vi "NavX.vi"(8 "error in":errorcluster) -> ()   [LabVIEW 2015]
uses:
  navx-mxp/labview/navX-MXP Library/COMMON/TypeDefs/Data TypeDefs/navX YPRH Data.ctl
  navx-mxp/labview/navX-MXP Library/COMMON/TypeDefs/Value TypeDefs/navX Interface Protocol.ctl
  <vilib>/Rock Robotics/SystemInterfaces/i2clib/i2c_bus.ctl
  LED Lights/LED Lights Global.vi
  <vilib>/Rock Robotics/Network Tables/NT Write Number.vi
  navx-mxp/labview/navX-MXP Library/navX-MXP IMU.lvlib
panel:
  out "Yaw":dbl
  out "YPRH":T1
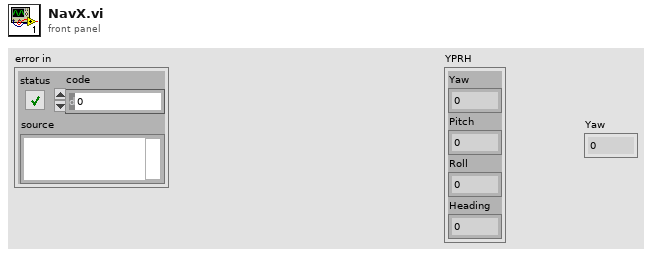
[diagram p1: front panel]
types:
  T1 = typedef "navX-MXP IMU.lvlib/navX YPRH Data.ctl" = cluster{"Yaw":dbl, "Pitch":dbl, "Roll":dbl, "Heading":dbl}
  T2 = typedef "i2c_bus.ctl" = enum16{"I2C On-Board", "I2C MXP", "Invalid"}
  T3 = typedef "navX-MXP IMU.lvlib/navX Interface Protocol.ctl" = enum16{"SPI", "I2C", "SERIAL"}
  T4 = typedef "NavX Light Global Type Def.ctl" = cluster{"NavX Error":errorcluster, "Initialized":bool}
  T5 = typedef "navX-MXP IMU.lvlib/navX Device TypeDef.ctl" = cluster{"navX Interface Protocol":T3, "navX Interface Protocol TypeDefs":cluster{"SPIDevRef":T6, "I2CDevRef":T8}, "navX System Information":cluster{"Board Information":T9, "Status":T12, "Offsets":T16, "LastSampleTimestamp":dbl, "LastSampleValid":bool}, "navX Common Information":cluster{"Update Rate (4Hz-60Hz)":T17, "refnum name":string, "error":errorcluster, "LastSampleFPGATimestamp":dbl}}
  T6 = typedef "WPI_SPIDevRef.ctl" = cluster{"DevStatus":errorcluster, "Handle":i32, "SPI Bus":T7}
  T7 = typedef "spi_bus.ctl" = enum16{"SPI On-Board, CS0", "SPI On-Board, CS1", "SPI On-Board, CS2", "SPI On-Board, CS3", "SPI MXP", "Invalid"}
  T8 = typedef "WPI_I2CDevRef.ctl" = cluster{"DevStatus":errorcluster, "Device Address":u8, "Handle":i32, "I2C Bus":T2}
  T9 = typedef "navX-MXP IMU.lvlib/navX Board Information.ctl" = cluster{"WhoAmI (50 | 0x32)":u8, "Board Revision":u8, "Firmware Major Version":u8, "Firmware Minor Version":u8, "NAVX_BOARD_CAPABILITY":T10, "NAVX_BOARD_YAW_AXIS":T11}
  T10 = typedef "navX-MXP IMU.lvlib/navX NAVX_BOARD_CAPABILITY.ctl" = cluster{"OMNIMOUNT":bool, "YAW_RESET":bool, "VEL_AND_DISP":bool}
  T11 = typedef "navX-MXP IMU.lvlib/navX NAVX_BOARD_YAW_AXIS.ctl" = cluster{"BOARD_YAW_AXIS_UP":bool, "BOARD_YAW_AXIS":u8}
  T12 = typedef "navX-MXP IMU.lvlib/navX Status Data.ctl" = cluster{"Update Rate Hz":u8, "Accelerometer Full-Scale Range":u8, "Gyro Full-Scale Range":u16, "NAVX_OP_STATUS":T13, "NAVX_CAL_STATUS":T14, "NAVX_SELFTEST_STATUS":u8, "NAVX_SENSOR_STATUS":T15}
  T13 = typedef "navX-MXP IMU.lvlib/navX NAVX_OP_STATUS.ctl" = u8
  T14 = typedef "navX-MXP IMU.lvlib/navX NAVX_CAL_STATUS.ctl" = u8
  T15 = typedef "navX-MXP IMU.lvlib/navX NAVX_SENSOR_STATUS.ctl" = cluster{"MOVING":bool, "YAW_STABLE":bool, "MAG_DISTURBANCE":bool, "ALTITUDE_VALID":bool, "SEALEVEL_PRESS_SET":bool, "FUSED_HEADING_VALID":bool}
  T16 = typedef "navX-MXP IMU.lvlib/navX Offsets Data.ctl" = cluster{"Yaw":dbl, "Quat W":dbl, "Quat X":dbl, "Quat Y":dbl, "Quat Z":dbl}
  T17 = typedef "navX-MXP IMU.lvlib/navX Update Rate.ctl" = u8
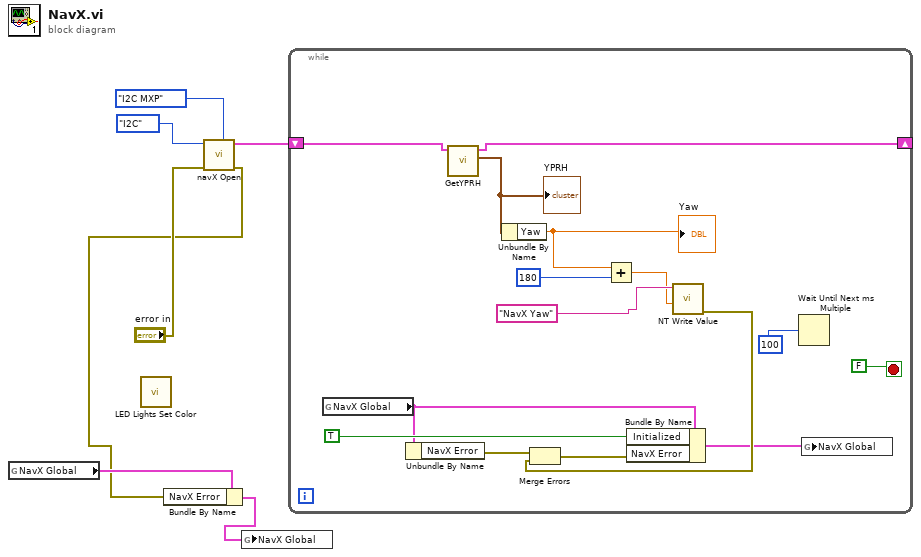
[diagram p0: block diagram]
diagram:
  n1 = global read "LED Lights Global.vi" "NavX Global"() -> (w3:T4)
  n2 = call "LED Lights Set Color.vi"() -> ()  [unwired: 10 in, 2 out]
  n3 = call "navX Open.vi"("I2C Bus"=i2c_bus."I2C MXP", "error in"="error in", "navX Interface Protocol"=navX_Interface_Protocol."I2C") -> ("error out"=w1:errorcluster, "navX Device TypeDef"=w7:T5)  [unwired: 6 in, 1 out]
  n4 = Bundle By Name(cluster=w3, "NavX Error"=w1) -> (w2:T4)
  n5 = global write "LED Lights Global.vi" "NavX Global"(w2) -> ()
  n6 = while {
    shift-right: [w19] -> _
    shift-left: w7 -> [w20]
    stop <- FALSE stop-if-true
    n7 = global read "LED Lights Global.vi" "NavX Global"() -> (w10:T4)
    n8 = Unbundle By Name(w10) -> ("NavX Error"=w8:errorcluster)
    n9 = call "GetYPRH.vi"("navX Device TypeDef"=w20) -> ("YPRH"=w18:T1, "navX Device TypeDef"=w19:T5)  [unwired: 8 in, 1 out]
    "YPRH" <- w18
    n10 = Unbundle By Name(w18) -> ("Yaw"=w16:dbl)
    "Yaw" <- w16
    n11 = Add(x=w16, y=180) -> (x+y=w14:dbl)
    n12 = call-poly <vilib>:"NT Write Value.vi"("Numeric"=w14, "Name"="NavX Yaw") -> ("error out"=w11:errorcluster)  [unwired: 9 in]
    n13 = Merge Errors(w8, w11) -> (w12:errorcluster)
    n14 = Bundle By Name(cluster=w10, "Initialized"=TRUE, "NavX Error"=w12) -> (w9:T4)
    n15 = Wait Until Next ms Multiple(millisecond multiple=u32 100) -> ()  [unwired: 1 out]
    n16 = global write "LED Lights Global.vi" "NavX Global"(w9) -> ()
  }
